vi "ex03_ITEM.vi"() -> ()   [LabVIEW 2011]
panel:
  in  "stop":bool
  out "Boolean 3":bool
  out "Boolean 2":bool
  in  "Boolean":bool
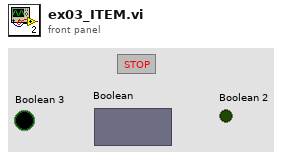
[diagram p1: front panel]
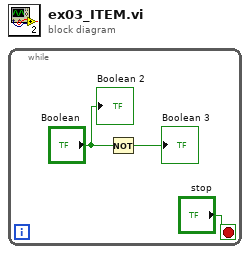
[diagram p0: block diagram]
diagram:
  n1 = while {
    stop <- "stop" stop-if-true
    n2 = Not(x="Boolean") -> (.not. x?=→"Boolean 3":bool)
    "Boolean 2" <- "Boolean"
  }
